vi "Is Window Being Shown (library variable).vi"() -> ()   [LabVIEW 2023, in "Error Manager.lvlib" / "New Error Window.lvlib"]
uses:
  New Error Window.lvlib
panel:
  out "Is Window Being Shown?":bool
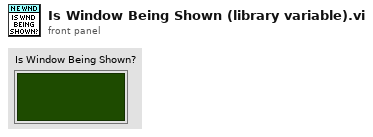
[diagram p1: front panel]
diagram:
